vi "_Disconnect_DB.vi"(8 "error in (no error)":errorcluster, 11 "Postgres Connector In":refnum<class "Postgres Connector.lvclass">) -> (0 "error out":errorcluster, 3 "Postgres Connector Out":refnum<class "Postgres Connector.lvclass">)   [LabVIEW 2020, in "Postgres Connector.lvclass"]
doc: "This VI is used to disconnect the user from the database"
uses:
  Postgres Connector.lvclass
  Postgres Connector.lvclass/Postgres Connector.ctl
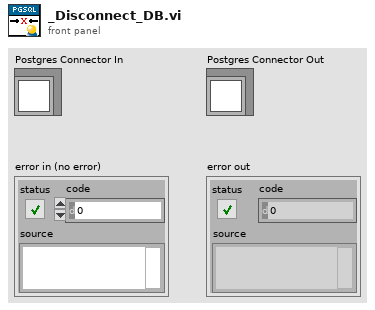
[diagram p1: front panel]
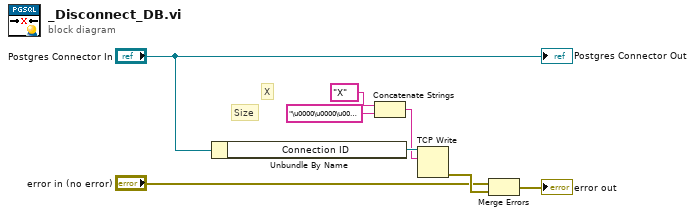
[diagram p0: block diagram]
diagram:
  # "Size"
  # "X"
  n1 = Unbundle By Name("Postgres Connector In") -> ("Connection ID"=w6:refnum<k5>)
  n2 = Concatenate Strings("X", "\u0000\u0000\u0000\u0004" ("string")) -> (w5:string)
  n3 = TCP Write(connection ID=w6, data in=w5) -> (error out=w8:errorcluster)  [unwired: 2 in, 2 out]
  n4 = Merge Errors("error in (no error)", w8) -> (→"error out":errorcluster)
  "Postgres Connector Out" <- "Postgres Connector In"
